vi "Check if Axis Selected.vi"(8 "error in (no error)":errorcluster, 11 "Cluster in":refnum<vi>) -> (0 "error out":errorcluster, 3 "Axis Selected":bool)   [LabVIEW 2014]
uses:
  <resource>/objmgr/nimcca.rc
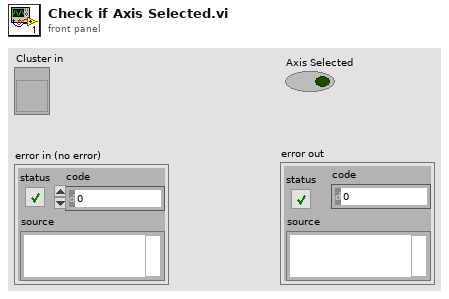
[diagram p1: front panel]
types:
  T1 = cluster{"Available Drives":i32, "Boolean":bool, "Path to Open.vi not listed (Optional)":path, "Axis":refnum<k21>}
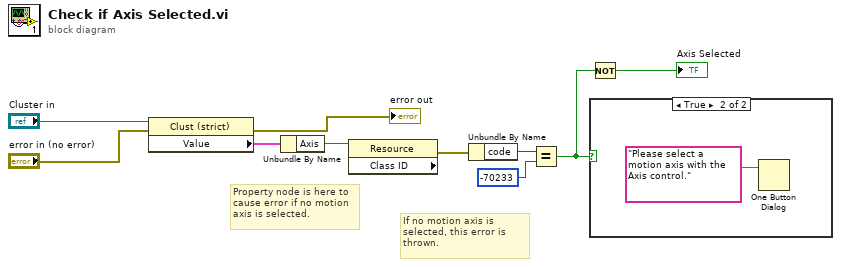
[diagram p0: block diagram]
diagram:
  # "If no motion axis is selected, this error is thrown."
  # "Property node is here to cause error if no motion axis is selected."
  n1 = property class="Clust (strict)"(reference="Cluster in", error in="error in (no error)") -> (error out=→"error out":errorcluster, "Value"=w5:T1)  [unwired: 1 out]
  n2 = Unbundle By Name(w5) -> ("Axis"=w4:refnum<k21>)
  n3 = property class="Resource" props=["Class ID"](reference=w4) -> (error out=w8:errorcluster)  [unwired: 1 in, 2 out]
  n4 = Unbundle By Name(w8) -> ("code"=w7:i32)
  n5 = Equal?(x=w7, y=-70233) -> (x = y?=w9:bool)
  n6 = Not(x=w9) -> (.not. x?=→"Axis Selected":bool)
  n7 = case shown="True" w9 {
    frame False {
    }
    frame True {
      n8 = One Button Dialog(message="Please select a motion axis with the Axis control.") -> ()  [unwired: 1 in, 1 out]
    }
  }
